vi "Insert Results into Excel.vi"(0 "report in":refnum<class "NI_report.lvclass">, 1 "strings":string[](array[string]), 2 "Pass/Fail":bool[](array[boolean]), 5 "column":i32, 7 "row":i32, 11 "error in":errorcluster) -> (4 "report out":refnum<class "NI_report.lvclass">, 6 "column out":i32, 15 "error out":errorcluster)   [LabVIEW 2015]
uses:
  SupportVIs/NI_report.lvclass
  SupportVIs/Append Report Text (str wrap).vi
  SupportVIs/NI_Excel.lvclass
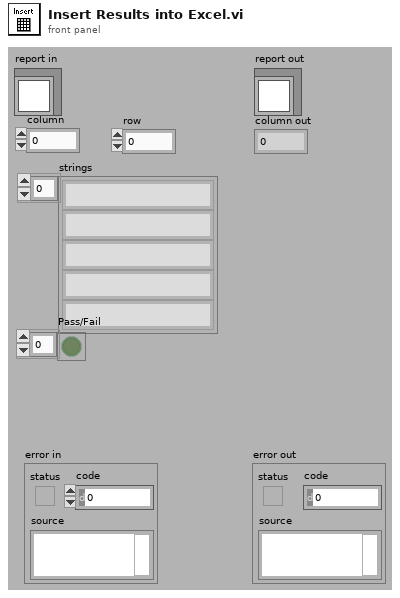
[diagram p1: front panel]
types:
  T1 = cluster{"position (excel)":cluster{"row":i32, "column":i32}, "name (excel)":string, "bookmark (word)":string}
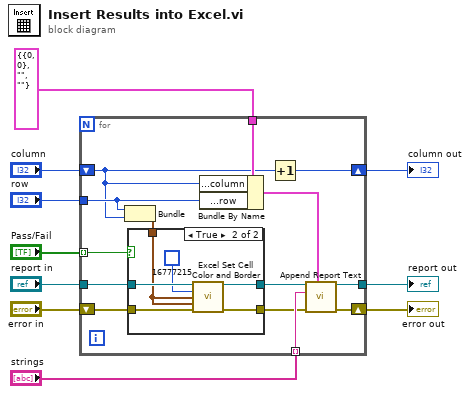
[diagram p0: block diagram]
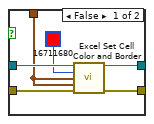
[diagram p2: hidden frame]
diagram:
  n1 = for {
    tunnel: "strings" -> [w24] mode=indexing
    tunnel: "report in" -> [w11]
    tunnel: [w23] -> w2
    shift-right: [w19] -> w5
    shift-left: "column" -> [w13]
    tunnel: T1 {"position (excel)"={"row"=0, "column"=0}, "name (excel)"="", "bookmark (word)"=""} ("MS Office parameters") -> [w21]
    tunnel: "row" -> [w16]
    shift-right: [w22] -> w1
    shift-left: "error in" -> [w12]
    tunnel: "Pass/Fail" -> [w14] mode=indexing
    n2 = Bundle("row"=w16, "column"=w13) -> (w15:cluster{"row":i32, "column":i32})  [unwired: 1 in]
    n3 = case shown="True" w14 {
      tunnel: [w30 w36] -> w18
      tunnel: [w29 w35] -> w17
      tunnel: w11 -> [w28 w34]
      tunnel: w12 -> [w27 w33]
      tunnel: w15 -> [w26 w32]
      frame False {
        n4 = call "Excel Set Cell Color and Border.vi"("report in"=w28, "background color (w)"=u32 16711680, "start (-1, -1)"=w26, "end (-1, -1)"=w26, "error in (no error)"=w27) -> ("report out"=w30:refnum<class "NI_report.lvclass">, "error out"=w29:errorcluster)  [unwired: 9 in]
      }
      frame True {
        n5 = call "Excel Set Cell Color and Border.vi"("report in"=w34, "background color (w)"=u32 16777215, "start (-1, -1)"=w32, "end (-1, -1)"=w32, "error in (no error)"=w33) -> ("report out"=w36:refnum<class "NI_report.lvclass">, "error out"=w35:errorcluster)  [unwired: 9 in]
      }
    }
    n6 = Bundle By Name(cluster=w21, "position (excel).column"=w13, "position (excel).row"=w16) -> (w20:T1)
    n7 = Increment(x=w13) -> (x+1=w19:i32)
    n8 = call-poly "Append Report Text.vi"("report in"=w18, "MS Office parameters"=w20, "text"=w24, "error in (no error)"=w17) -> ("report out"=w23:refnum<class "NI_report.lvclass">, "error out"=w22:errorcluster)  [unwired: 8 in, 2 out]
  }
  "error out" <- w1
  "column out" <- w5
  "report out" <- w2
